vi "create.grid.vi"(9 "Draw Area Size":T1, 10 "Plot End":timestamp, 11 "Plot Start":timestamp) -> (3 "picture":picture)   [LabVIEW 2024]
uses:
  <vilib>/Utility/miscctls.llb/LVBoundsTypeDef.ctl
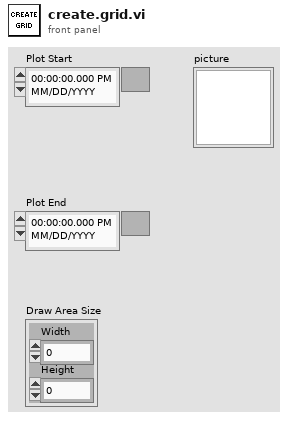
[diagram p1: front panel]
types:
  T1 = typedef "LVBoundsTypeDef.ctl" = cluster{"Width":u32, "Height":u32}
  T2 = cluster{"Width":u16, "Style":enum32{"Solid", "Dash", "Dot", "DashDot", "DashDotDot"}}
  T3 = enum16{"None", "Stacked", "Clockwise", "Counterclockwise"}
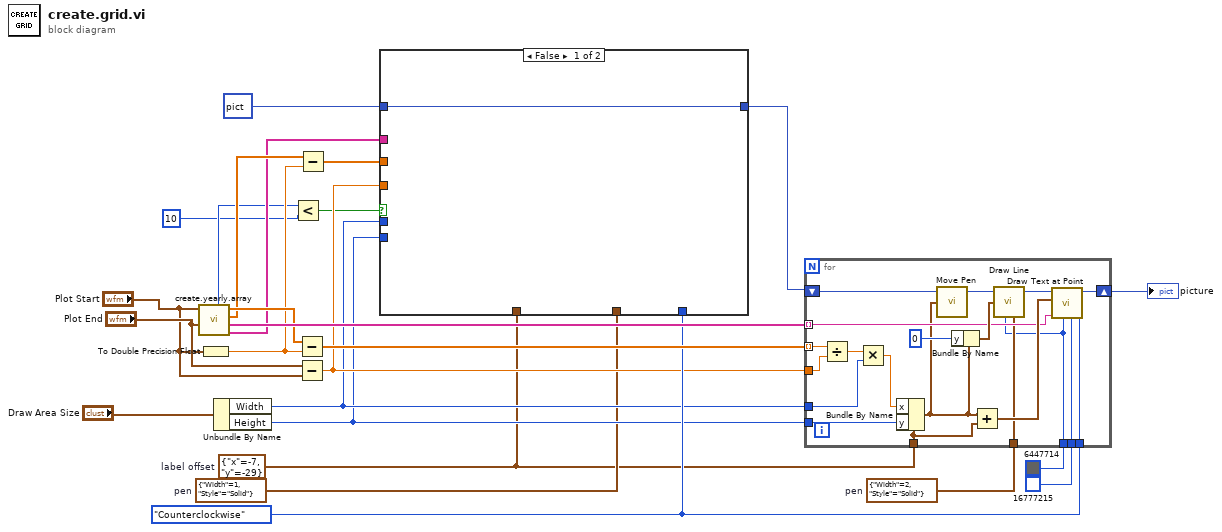
[diagram p0: block diagram]
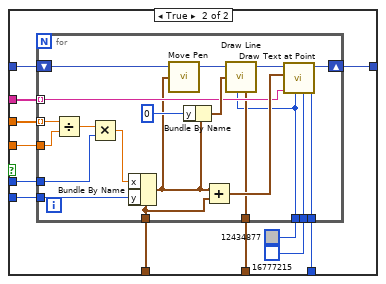
[diagram p2: hidden frame]
diagram:
  w1 = T2 {"Width"=2, "Style"=enum."Solid"}  # pen
  w6 = T2 {"Width"=1, "Style"=enum."Solid"}  # pen
  w16 = T3."Counterclockwise" ("text orientation")
  w5 = cluster{"x":i16, "y":i16} {"x"=-7, "y"=-29}  # label offset
  n1 = call "create.yearly.array.vi"("end time"="Plot End", "start time"="Plot Start") -> ("month_names"=w10:string[], "year_names"=w20:string[], "month_timestamps"=w12:dbl[], "year_timestamps"=w17:dbl[], "years"=w4:i32)  [unwired: 5 in]
  n2 = To Double Precision Float(number="Plot Start") -> (double precision float=w11:dbl)
  n3 = Unbundle By Name("Draw Area Size") -> ("Width"=w8:u32, "Height"=w7:u32)
  n4 = Less?(x=w4, y=10) -> (x < y?=w2:bool)
  n5 = Subtract(x=w17, y=w11) -> (x-y=w18:dbl[])
  n6 = Subtract(x="Plot End", y="Plot Start") -> (x-y=w9:dbl)
  n7 = Subtract(x=w12, y=w11) -> (x-y=w13:dbl[])
  n8 = case shown="False" w2 {
    tunnel: w16 -> [_ w38]
    tunnel: [w26 w37] -> w15
    tunnel: picture data[5B] ("picture") -> [w26 w36]
    tunnel: w13 -> [_ w35]
    tunnel: w10 -> [_ w34]
    tunnel: w9 -> [_ w33]
    tunnel: w8 -> [_ w32]
    tunnel: w7 -> [_ w31]
    tunnel: w6 -> [_ w28]
    tunnel: w5 -> [_ w27]
    frame False {
    }
    frame True {
      n9 = for {
        tunnel: w35 -> [w58] mode=indexing
        shift-right: [w51] -> w37
        shift-left: w36 -> [w50]
        tunnel: w33 -> [w57]
        tunnel: w32 -> [w55]
        tunnel: w31 -> [w54]
        tunnel: w34 -> [w46] mode=indexing
        tunnel: w38 -> [w45]
        tunnel: w28 -> [w44]
        tunnel: w27 -> [w41]
        tunnel: u32 16777215 ("BG color(transparent)") -> [w42]
        tunnel: u32 12434877 ("color(black)") -> [w40]
        n10 = Divide(x=w58, y=w57) -> (x/y=w56:dbl)
        n11 = Multiply(x=w56, y=w55) -> (x*y=w39:dbl)
        n12 = Bundle By Name(cluster=w41, "x"=w39, "y"=w54) -> (w43:cluster{"x":i16, "y":i16})
        n13 = call <vilib>:"Move Pen.vi"("new position"=w43, "picture"=w50) -> ("new picture"=w53:picture)  [unwired: 3 in]
        n14 = Bundle By Name(cluster=w43, "y"=i16 0) -> (w47:cluster{"x":i16, "y":i16})
        n15 = Add(x=w43, y=w41) -> (x+y=w49:cluster{"x":i16, "y":i16})
        n16 = call <vilib>:"Draw Line.vi"("picture"=w53, "end point"=w47, "color(black)"=w40, "pen"=w44) -> ("new picture"=w52:picture)  [unwired: 5 in]
        n17 = call <vilib>:"Draw Text at Point.vi"("text orientation"=w45, "BG color(transparent)"=w42, "text color(black)"=w40, "text"=w46, "origin"=w49, "picture"=w52) -> ("new picture"=w51:picture)  [unwired: 4 in, 1 out]
      }
    }
  }
  n18 = for {
    tunnel: w18 -> [w78] mode=indexing
    shift-right: [w71] -> w21
    shift-left: w15 -> [w70]
    tunnel: w9 -> [w77]
    tunnel: w8 -> [w75]
    tunnel: w7 -> [w74]
    tunnel: w20 -> [w66] mode=indexing
    tunnel: w16 -> [w65]
    tunnel: w1 -> [w64]
    tunnel: w5 -> [w61]
    tunnel: u32 16777215 ("BG color(transparent)") -> [w62]
    tunnel: u32 6447714 ("color(black)") -> [w60]
    n19 = Divide(x=w78, y=w77) -> (x/y=w76:dbl)
    n20 = Multiply(x=w76, y=w75) -> (x*y=w59:dbl)
    n21 = Bundle By Name(cluster=w61, "x"=w59, "y"=w74) -> (w63:cluster{"x":i16, "y":i16})
    n22 = call <vilib>:"Move Pen.vi"("new position"=w63, "picture"=w70) -> ("new picture"=w73:picture)  [unwired: 3 in]
    n23 = Bundle By Name(cluster=w63, "y"=i16 0) -> (w67:cluster{"x":i16, "y":i16})
    n24 = Add(x=w63, y=w61) -> (x+y=w69:cluster{"x":i16, "y":i16})
    n25 = call <vilib>:"Draw Line.vi"("picture"=w73, "end point"=w67, "color(black)"=w60, "pen"=w64) -> ("new picture"=w72:picture)  [unwired: 5 in]
    n26 = call <vilib>:"Draw Text at Point.vi"("text orientation"=w65, "BG color(transparent)"=w62, "text color(black)"=w60, "text"=w66, "origin"=w69, "picture"=w72) -> ("new picture"=w71:picture)  [unwired: 4 in, 1 out]
  }
  "picture" <- w21
